vi "ASDTCPDemo.vi"() -> ()   [LabVIEW 2010]
uses:
  Instance           9 18Saved   ASDTCPDemo .vi
panel:
  out "Complete":bool
  out "Error Description":string
  out "Header Description":string
  out "Reflectance Spectrum":dbl[](graph)
  out "Dark Corrected Spectrum":dbl[](graph)
  out "VNIR Integration Time":string
  out "Header Code":i32
  out "Error Code":i32
  out "Swir 2 Offset":i32
  out "Swir 2 Gain":i32
  out "Swir 1 Offset":i32
  out "Swir 1 Gain":i32
  out "VNIR Integration Code":i32
  out "Ending Wavelength":dbl
  out "Starting Wavelength":dbl
  out "Acquired Spectrum":sgl[](graph)
  in  "Send Command":bool
  in  "Command":u16(ring) items=["Acquire Spectrum", "Read Starting Wavelength", "Read Ending Wavelength", "Optimize", "Acquire Dark Corrected Spectrum", "Acquire a Reflectance Spectrum", "Restore"]
  in  "stop":bool
  # "Instructions:\n1.  Run this app \n2. Specify the IP address of the ASD instrument, which is 169.254.1.11    After a connection is made, issue the \"Restore\" command.\n3. Select a command type and press 'Send Command'. \n4. Allow command to complete before pressing  'Stop'"
  # "ASD TCP Demo Version 2.0"
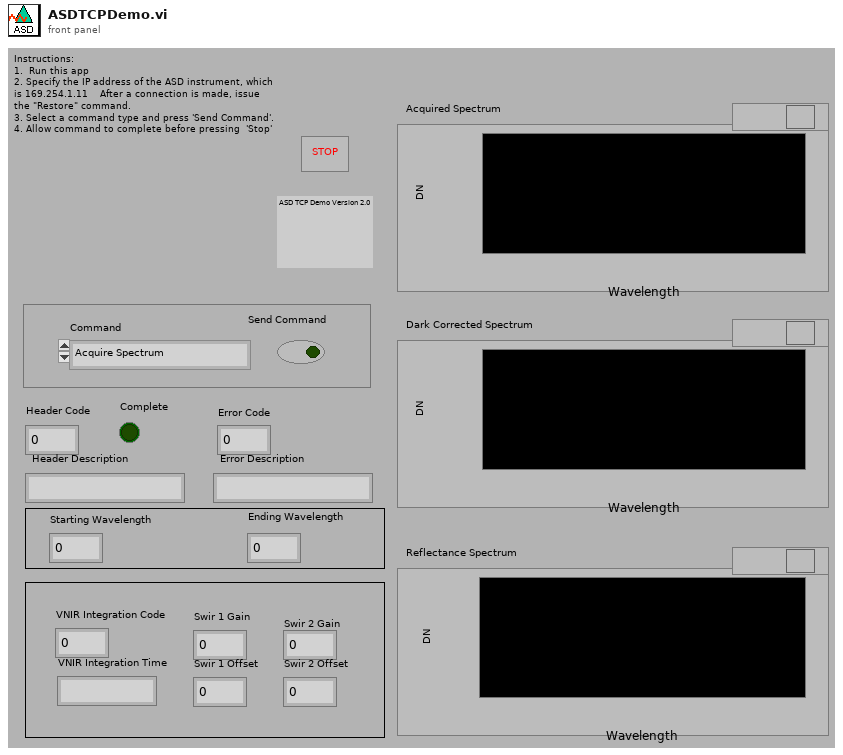
[diagram p1: front panel]
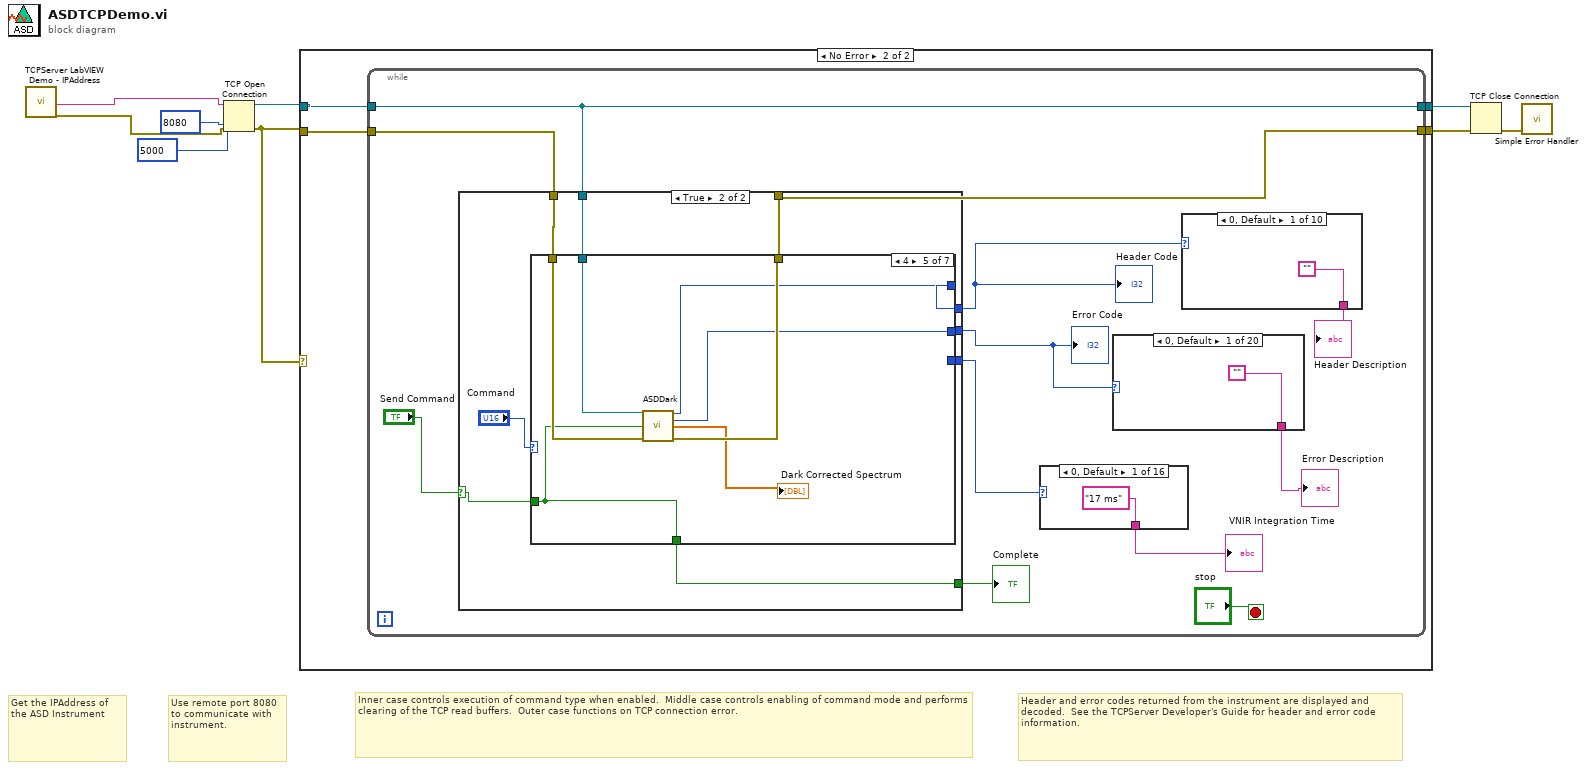
[diagram p0: block diagram]
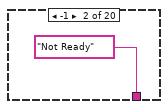
[diagram p3: hidden frame]
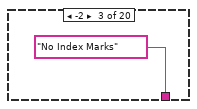
[diagram p4: hidden frame]
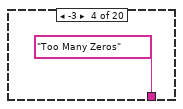
[diagram p5: hidden frame]
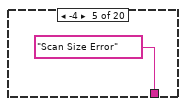
[diagram p6: hidden frame]
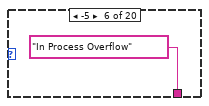
[diagram p7: hidden frame]
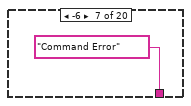
[diagram p8: hidden frame]
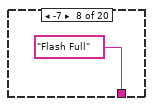
[diagram p9: hidden frame]
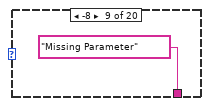
[diagram p10: hidden frame]
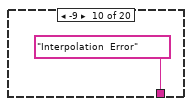
[diagram p11: hidden frame]
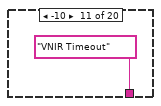
[diagram p12: hidden frame]
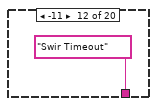
[diagram p13: hidden frame]
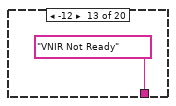
[diagram p14: hidden frame]
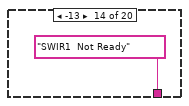
[diagram p15: hidden frame]
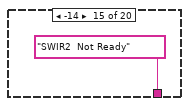
[diagram p16: hidden frame]
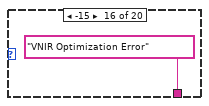
[diagram p17: hidden frame]
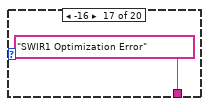
[diagram p18: hidden frame]
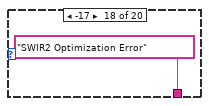
[diagram p19: hidden frame]
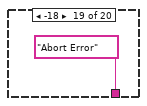
[diagram p20: hidden frame]
diagram:
  # "Get the IPAddress of the ASD Instrument"
  # "Header and error codes returned from the instrument are displayed and decoded.  See the TCPServer Developer's Guide for header and error code information."
  # "Inner case controls execution of command type when enabled.  Middle case controls enabling of command mode and performs clearing of the TCP read buffers.  Outer case functions on TCP connection error."
  # "Use remote port 8080  to communicate with instrument."
  n1 = call "TCPServer LabVIEW Demo - IPAddress"() -> ("IPAddress"=w2:string, "error out"=w1:errorcluster)  [unwired: 17 in, 1 out]
  n2 = TCP Open Connection(address=w2, remote port or service name=u16 8080 ("local port"), timeout ms (60000)=u16 5000 ("remote port"), error in (no error)=w1) -> (connection ID=w9:refnum<k5>, error out=w3:errorcluster)  [unwired: 1 in]
  n3 = case shown="No Error" w3 {
    tunnel: w9 -> [w10 w15]
    tunnel: [w10 w14] -> w8
    tunnel: [w11 w13] -> w7
    tunnel: w3 -> [w11 w12]
    frame Error {
    }
    frame No Error {
      n4 = while {
        tunnel: w15 -> [w24]
        tunnel: [w24] -> w14
        tunnel: [w25] -> w13
        tunnel: w12 -> [w26]
        stop <- "stop" stop-if-true
        n5 = case shown="True" "Send Command" {
          selector: "Send Command" -> [_ w87]
          tunnel: w26 -> [w76 w90]
          tunnel: [w76 w89] -> w25
          tunnel: w24 -> [w82 w88]
          tunnel: [_ w86] -> w21
          tunnel: [_ w85] -> w19
          tunnel: [_ w84] -> w23
          tunnel: [FALSE w83] -> w16
          frame False {
            # "When the instrument first makes the TCP Connection, it sends system and version information.  This operation clear this data from the TCP receive buffer.  It also verifys the receive buffer is cleared between commands."
            n6 = TCP Write(connection ID=w82, data in="", error in (no error)=w76) -> (connection ID out=w81:refnum<k5>, error out=w80:errorcluster)  [unwired: 1 in, 1 out]
            n7 = TCP Read(connection ID=w81, bytes to read=100, error in (no error)=w80, 9:1000 ("timeout ms (25000)")) -> (error out=w75:errorcluster)  [unwired: 1 in, 2 out]
            n8 = call <vilib>:"Clear Errors.vi"("error in (no error)"=w75) -> ()  [unwired: 6 in, 1 out]
          }
          frame True {
            n9 = case shown="4" "Command" {
              tunnel: w90 -> [w98 w105 w112 w123 w130 w137 w143]
              tunnel: [w97 w104 w111 w116 w129 w136 w142] -> w89
              tunnel: w88 -> [w96 w103 w110 w122 w128 w135 w138]
              tunnel: w87 -> [w92 w99 w106 w113 w124 w131 w141]
              tunnel: [w95 w100 w109 w121 w127 w134 w140] -> w86
              tunnel: [w94 w101 w108 w120 w126 w133 w139] -> w85
              tunnel: [_ _ _ w114 _ _ _] -> w84
              tunnel: [w92 w99 w106 w113 w124 w131 w141] -> w83
              frame 0, Default {
                n10 = call "ASDAcquire.vi"("TCP Network Connection Refnum"=w96, "Acquire"=w92, "error in (no error)"=w98) -> ("Header Code"=w95:i32, "Error Code"=w94:i32, "Spectrum Data"=→"Acquired Spectrum":sgl[], "error out"=w97:errorcluster)  [unwired: 9 in]
              }
              frame 1 {
                n11 = call "ASDStartingWavelength.vi"("TCP Network Connection Refnum"=w103, "Get Starting Wavelength"=w99, "error in (no error)"=w105) -> ("Header Code"=w100:i32, "Error Code"=w101:i32, "Starting Wavelength"=→"Starting Wavelength":dbl, "error out"=w104:errorcluster)  [unwired: 9 in]
              }
              frame 2 {
                n12 = call "ASDEndingWavelength.vi"("TCP Network Connection Refnum"=w110, "Get Ending Wavelength"=w106, "error in (no error)"=w112) -> ("Header Code"=w109:i32, "Error Code"=w108:i32, "Ending Wavelength"=→"Ending Wavelength":dbl, "error out"=w111:errorcluster)  [unwired: 9 in]
              }
              frame 3 {
                n13 = call "ASDOptimize.vi"("TCP Network Connection Refnum"=w122, "Optimize"=w113, "error in (no error)"=w123) -> ("Header Code"=w121:i32, "Error Code"=w120:i32, "VNIR Integration Time"=w114:i32, "SWIR 1 Gain"=→"Swir 1 Gain":i32, "SWIR 2 Gain"=→"Swir 1 Offset":i32, "SWIR 1 Offset"=→"Swir 2 Offset":i32, "SWIR 2 Offset"=→"Swir 2 Gain":i32, "error out"=w116:errorcluster)  [unwired: 17 in]
                "VNIR Integration Code" <- w114
              }
              frame 4 {
                n14 = call "ASDDark.vi"("TCP Network Connection Refnum"=w128, "Collect Dark"=w124, "error in (no error)"=w130) -> ("Header Code"=w127:i32, "Error Code"=w126:i32, "Dark Corrected Spectrum Data"=→"Dark Corrected Spectrum":dbl[], "error out"=w129:errorcluster)  [unwired: 9 in]
              }
              frame 5 {
                n15 = call "ASDReflectance.vi"("TCP Network Connection Refnum"=w135, "Collect Reflectance Spectrum"=w131, "error in (no error)"=w137) -> ("Header Code"=w134:i32, "Error Code"=w133:i32, "Reflectance Spectrum"=→"Reflectance Spectrum":dbl[], "error out"=w136:errorcluster)  [unwired: 9 in]
              }
              frame 6 {
                n16 = call "ASDRestore.vi"("TCP Network Connection Refnum"=w138, "Restore Flash"=w141, "error in (no error)"=w143) -> ("Header Code"=w140:i32, "Error Code"=w139:i32, "error out"=w142:errorcluster)  [unwired: 10 in]
              }
            }
          }
        }
        "Error Code" <- w19
        "Header Code" <- w21
        "Complete" <- w16
        n17 = case shown="0, Default" w23 {
          tunnel: ["17 ms" "34 ms" "68 ms" "136 ms" "272 ms" "544 ms" "1.088 s" "2.176 s" "4 s" "8 s" "17 s" "34 s" "69 s" "139 s" "278 s" "557 s"] -> w22
          frame 0, Default {
          }
          frame 1 {
          }
          frame 2 {
          }
          frame 3 {
          }
          frame 4 {
          }
          frame 5 {
          }
          frame 6 {
          }
          frame 7 {
          }
          frame 8 {
          }
          frame 9 {
          }
          frame 10 {
          }
          frame 11 {
          }
          frame 12 {
          }
          frame 13 {
          }
          frame 14 {
          }
          frame 15 {
          }
        }
        "VNIR Integration Time" <- w22
        n18 = case shown="0, Default" w19 {
          tunnel: ["" "Not Ready" ("Header Description") "No Index Marks" ("Header Description") "Too Many Zeros" ("Header Description") "Scan Size Error" ("Header Description") "In Process Overflow" ("Header Description") "Command Error" ("Header Description") "Flash Full" ("Header Description") "Missing Parameter" ("Header Description") "Interpolation  Error" ("Header Description") "VNIR Timeout" ("Header Description") "Swir Timeout" ("Header Description") "VNIR Not Ready" ("Header Description") "SWIR1  Not Ready" ("Header Description") "SWIR2  Not Ready" ("Header Description") "VNIR Optimization Error" ("Header Description") "SWIR1 Optimization Error" ("Header Description") "SWIR2 Optimization Error" ("Header Description") "Abort Error" ("Header Description") "Parameter Error" ("Header Description")] -> w18
          frame 0, Default {
          }
          frame -1 {
          }
          frame -2 {
          }
          frame -3 {
          }
          frame -4 {
          }
          frame -5 {
          }
          frame -6 {
          }
          frame -7 {
          }
          frame -8 {
          }
          frame -9 {
          }
          frame -10 {
          }
          frame -11 {
          }
          frame -12 {
          }
          frame -13 {
          }
          frame -14 {
          }
          frame -15 {
          }
          frame -16 {
          }
          frame -17 {
          }
          frame -18 {
          }
          frame -19 {
          }
        }
        "Error Description" <- w18
        n19 = case shown="0, Default" w21 {
          tunnel: ["" "No Error" ("Header Description") "Collect Error" ("Header Description") "Flash not Loaded" ("Header Description") "Init Error" ("Header Description") "Flash Error" ("Header Description") "Reset Error" ("Header Description") "Interpolate Error" ("Header Description") "Optimize Error" ("Header Description") "Instrument Control Error" ("Header Description")] -> w20
          frame 0, Default {
          }
          frame 100 {
          }
          frame 200 {
          }
          frame 300 {
          }
          frame 400 {
          }
          frame 500 {
          }
          frame 600 {
          }
          frame 700 {
          }
          frame 800 {
          }
          frame 900 {
          }
        }
        "Header Description" <- w20
      }
    }
  }
  n20 = TCP Close Connection(connection ID=w8, error in (no error)=w7) -> (error out=w6:errorcluster)  [unwired: 1 in, 1 out]
  n21 = call <vilib>:"Simple Error Handler.vi"("error in (no error)"=w6) -> ()  [unwired: 4 in, 5 out]
